vi "Open UI.vi"(11 "Process in":refnum<class "ABD.lvclass">) -> (0 "error out":errorcluster, 3 "Process out":refnum<class "ABD.lvclass">)   [LabVIEW 2021, in "ABD.lvlib" / "ABD.lvclass"]
uses:
  ABD.lvclass
  ABD.lvclass/ABD.ctl
  ABD Panel/Main Panel.vi
  LVCAM/LVCAM/LVCAM/LVCAM.lvclass
  ABD Panel/ABD Panel.lvclass
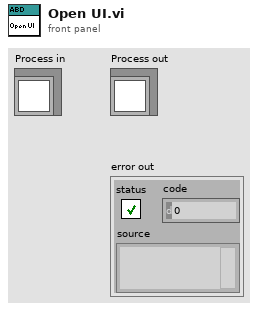
[diagram p1: front panel]
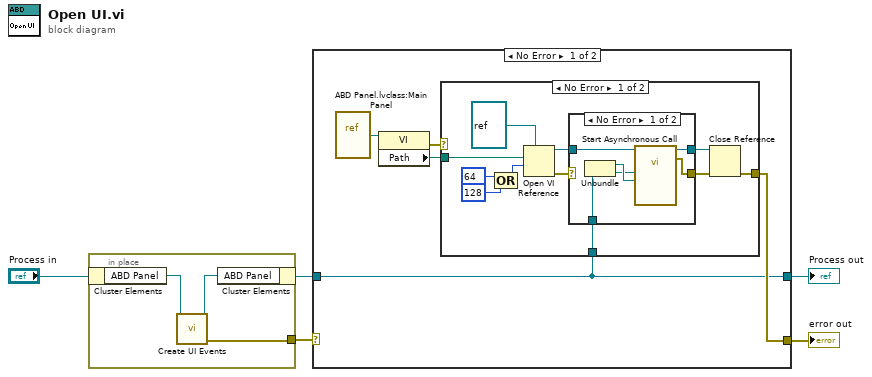
[diagram p0: block diagram]
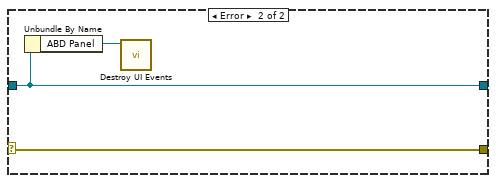
[diagram p4: hidden frame]
diagram:
  n1 = in-place {
    in-place-border: [w8] -> w1
    n2 = in-place-cluster #1("Process in") -> ("ABD Panel"=w6:refnum<class "ABD Panel.lvclass">)
    n3 = call "Create UI Events.vi"("ABD Panel in"=w6) -> ("error out"=w8:errorcluster, "ABD Panel out"=w7:refnum<class "ABD Panel.lvclass">)  [unwired: 9 in]
    n4 = in-place-cluster #1("ABD Panel"=w7) -> (w2:refnum<class "ABD.lvclass">)
  }
  n5 = case shown="No Error" w1 {
    selector: w1 -> [_ w36]
    tunnel: [w10 w36] -> w5
    tunnel: w2 -> [w9 w35]
    tunnel: [w9 w35] -> w4
    frame No Error {
      n6 = vi-ref "ABD Panel.lvclass:Main Panel.vi"() -> (w12:refnum<vi>)
      n7 = property class="VI"(reference=w12) -> (error out=w13:errorcluster, "Path"=w11:path)  [unwired: 1 in, 1 out]
      n8 = case shown="No Error" w13 {
        selector: w13 -> [_ w33]
        tunnel: [w22 w33] -> w10
        tunnel: w11 -> [w18 _]
        tunnel: w9 -> [w14 _]
        frame No Error {
          n9 = Compound Arithmetic op=OR(64 ("options: Multiple Clones,\n  Fire & Forget"), 128 ("options: Multiple Clones,\n  Fire & Forget")) -> (w20:i32)
          n10 = Open VI Reference(type specifier VI Refnum (for type only)=refnum<vi> refnum, vi path=w18, options=w20) -> (vi reference=w16:refnum<vi>, error out=w17:errorcluster)  [unwired: 3 in]
          n11 = case shown="No Error" w17 {
            selector: w17 -> [_ w32]
            tunnel: [w30 w31] -> w24
            tunnel: [w29 w32] -> w23
            tunnel: w16 -> [w28 w31]
            tunnel: w14 -> [w27 _]
            frame No Error {
              n12 = Unbundle(w27) -> (w26:refnum<class "LVCAM.lvclass">, w25:refnum<class "ABD Panel.lvclass">)
              n13 = call-by-ref "Start Asynchronous Call"(reference=w28, "LVCAM"=w26, "ABD Panel"=w25) -> (reference out=w30:refnum<vi>, error out=w29:errorcluster)  [unwired: 11 in]
            }
            frame Error {
            }
          }
          n14 = Close Reference(reference=w24, error in (no error)=w23) -> (error out=w22:errorcluster)
        }
        frame Error {
        }
      }
    }
    frame Error {
      n15 = Unbundle By Name(w35) -> ("ABD Panel"=w34:refnum<class "ABD Panel.lvclass">)
      n16 = call "Destroy UI Events.vi"("ABD Panel in"=w34) -> ()  [unwired: 11 in]
    }
  }
  "error out" <- w5
  "Process out" <- w4
